vi "Configure Control (Ring).vi"(8 "error in (no error)":errorcluster, 10 "control":refnum<vi>, 11 "NT Enum in":refnum<class "NT Enum.lvclass">) -> (0 "error out":errorcluster, 2 "control out":refnum<vi>, 3 "NT Enum out":refnum<class "NT Enum.lvclass">)   [LabVIEW 2020, in "PV Access.lvlib" / "PV Data.lvlib" / "NT Enum.lvclass"]
doc: "Set the description of <B>control</B> from the value's metadata."
uses:
  NT Enum.lvclass
  NT Enum.lvclass/NT Enum.ctl
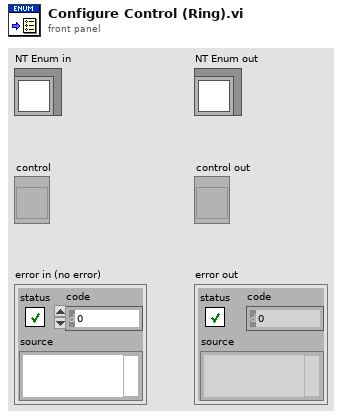
[diagram p1: front panel]
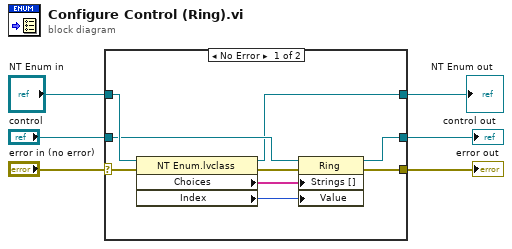
[diagram p0: block diagram]
diagram:
  n1 = case shown="No Error" "error in (no error)" {
    selector: "error in (no error)" -> [w15 w18]
    tunnel: [w12 w18] -> w5
    tunnel: "control" -> [w11 w17]
    tunnel: [w8 w17] -> w3
    tunnel: "NT Enum in" -> [w14 w16]
    tunnel: [w7 w16] -> w1
    frame No Error {
      n2 = property class="NT Enum.lvclass"(reference=w14, error in=w15) -> (reference out=w7:refnum<class "NT Enum.lvclass">, error out=w13:errorcluster, "Choices"=w10:string[], "Index"=w9:i32)
      n3 = property class="Ring"(reference=w11, error in=w13, "Strings []"=w10, "Value"=w9) -> (reference out=w8:refnum<vi>, error out=w12:errorcluster)
    }
    frame Error {
    }
  }
  "error out" <- w5
  "NT Enum out" <- w1
  "control out" <- w3
